vi "QTrkSetPixelCalibrationFactors.vi"(8 "error in (no error)":errorcluster, 9 "gainFactor (1)":sgl, 10 "offsetFactor (1)":sgl, 11 "QTrk Instance":T1) -> (0 "error out":errorcluster, 3 "QTrk Instance":T1)   [LabVIEW 2011]
uses:
  QTrkInstance.ctl
  QTrkDLL.vi
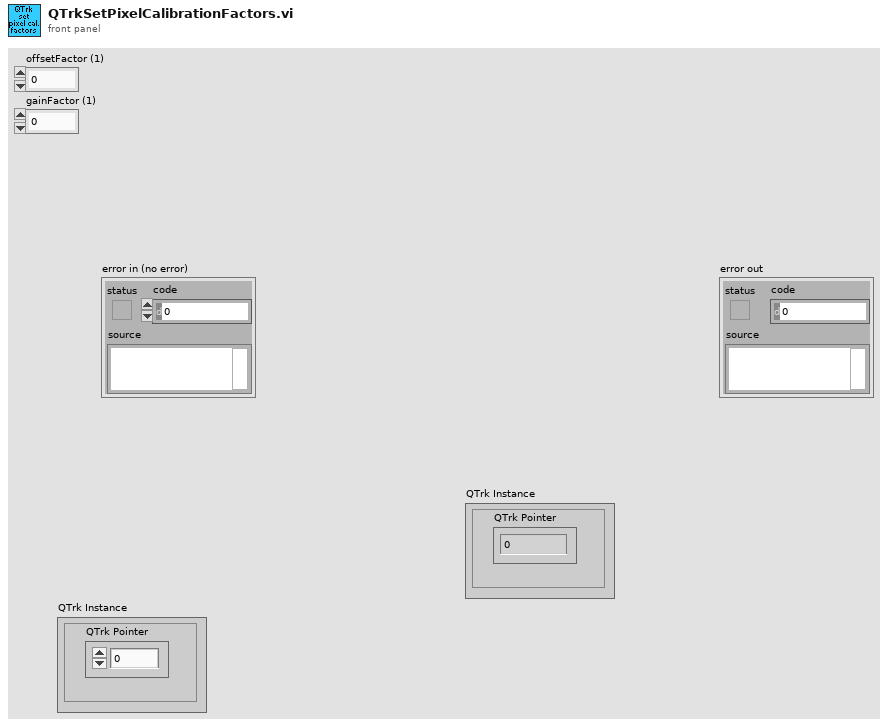
[diagram p1: front panel]
types:
  T1 = typedef "QTrkInstance.ctl" = cluster{"QTrk Pointer":u64}
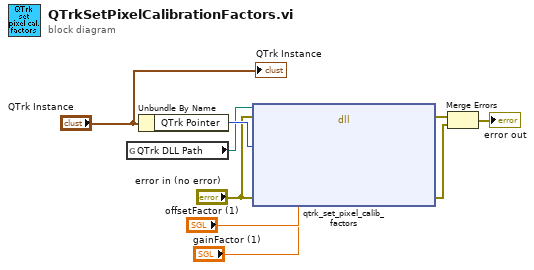
[diagram p0: block diagram]
diagram:
  n1 = global read "QTrkDLL.vi" "QTrk DLL Path"() -> (w7:path)
  n2 = Unbundle By Name("QTrk Instance") -> ("QTrk Pointer"=w8:u64)
  n3 = dll-call lib="D:/jcnossen1/cudaqi-tracker/bin/jtrk-labview.dll" fn="qtrk_set_pixel_calib_factors"(path in=w7, error in="error in (no error)", "tracker"=w8, "offsetFactor"="offsetFactor (1)", "gainFactor"="gainFactor (1)", "error"="error in (no error)") -> (error out=w6:errorcluster, "error"=w3:errorcluster)  [unwired: 5 in, 1 out]
  n4 = Merge Errors(w6, w3) -> (→"error out":errorcluster)
  "QTrk Instance" <- "QTrk Instance"
